vi "Extract IRF from PSED v2.vi"(6 "Termination Criteria":T1={"Max Iterations"=0, "Max Function Calls"=0, "Max Time"=1000.0, "Function Tolerance"=1e-06, "Parameter Tolerance"=1e-06, "Gradient Tolerance"=0.0, "Min Lambda"=1e-06, "Max Lambda"=1e-06, "Initial Tick Count"=0}, 8 "Error In":errorcluster, 9 "IRF*PSED Fixed Parameters":T7={"order"=0, "T"=0.0, "Time Constant Array"=[], "{S_k, C_k, phi_k, e_k} arrays"={"S_k Array"=[], "C_k Array"=[], "phi_k Array"=[], "e_k Array"=[]}, "IRF Extraction Options"={"Time Constant for IRF Extraction"=1e-18, "IRF Order"=0, "Fourier Series Smoothing"=enum."None", "Noise Threshold"=0.0, "Smoothing Width"=0.0, "Fourier Series Truncation"=enum."Automatic", "Truncation Order"=0, "Save Power Spectrum"=FALSE, "Smoothing"=FALSE, "Smoothing Parameter"=0.0, "Smoothing Order"=1, "Method"=enum."Direct"}} {"IRF Extraction Options"."Smoothing Order" min=1 max=10; "IRF Extraction Options"."Time Constant for IRF Extraction" format="%#_5g"}, 10 "Fit Settings":T2={"Use Original Plot # Points"=TRUE, "# Fit Plot Points"=0, "Fitting Method"=enum."Least Square", "Weighted Fit"=TRUE, "Show All Fit Components"=FALSE, "Axis Type"=0, "Show Fit Residuals"=TRUE, "Residual Type"=enum."Standard", "Fitting Algorithm"=enum."Levenberg-Marquardt"} {"Axis Type" items=["Linear", "Logarithmic"]}, 11 "Selected Plot Info":T12={"Multiplot XY Graph"=refnum, "Mouse Coordinates"={"Horizontal"=0, "Vertical"=0}, "Plot Index"=-1}) -> (0 "Error Out":errorcluster, 1 "Fit Result String":string, 2 "Power Spectrum":dbl[](array[numeric]), 3 "IRF Plot":cluster{"X Array":dbl[], "Y Array":dbl[]}, 5 "Smoothed Power Spectrum":dbl[](array[numeric]))   [LabVIEW 2021, in "Fits.lvlib"]
doc: "Extract IRF from provided decay and time constant"
uses:
  Fits.lvlib
  Graphs/XY Graph/XY Graph Selected Plot Info.ctl
  Graphs/XY Graph/XY Graph Refnum.ctl
  <vilib>/Utility/miscctls.llb/LVPoint32TypeDef.ctl
  IRF(X)PSED Fixed Parameters v3.ctl
  IRF(X)PSED Extraction Options.ctl
  Fourier Series Smoothing Option.ctl
  Fourier Series Truncation.ctl
  IRF Extraction Method.ctl
  Fit Settings.ctl
  Nonlinear Fit Method.ctl
  Ramp Type.ctl
  Residual Type.ctl
  Non-linear Fitting Algorithm.ctl
  My Fit Stopping Criteria.ctl
  Fit Plot Request Information.ctl
  <vilib>/Utility/miscctls.llb/LVPointDoubleTypeDef.ctl
  Fit Models.ctl
  D-Only Fixed Parameters.ctl
  Error/Error.lvlib
  Graphs/XY Graph/XY Graph Add-Ons.lvlib
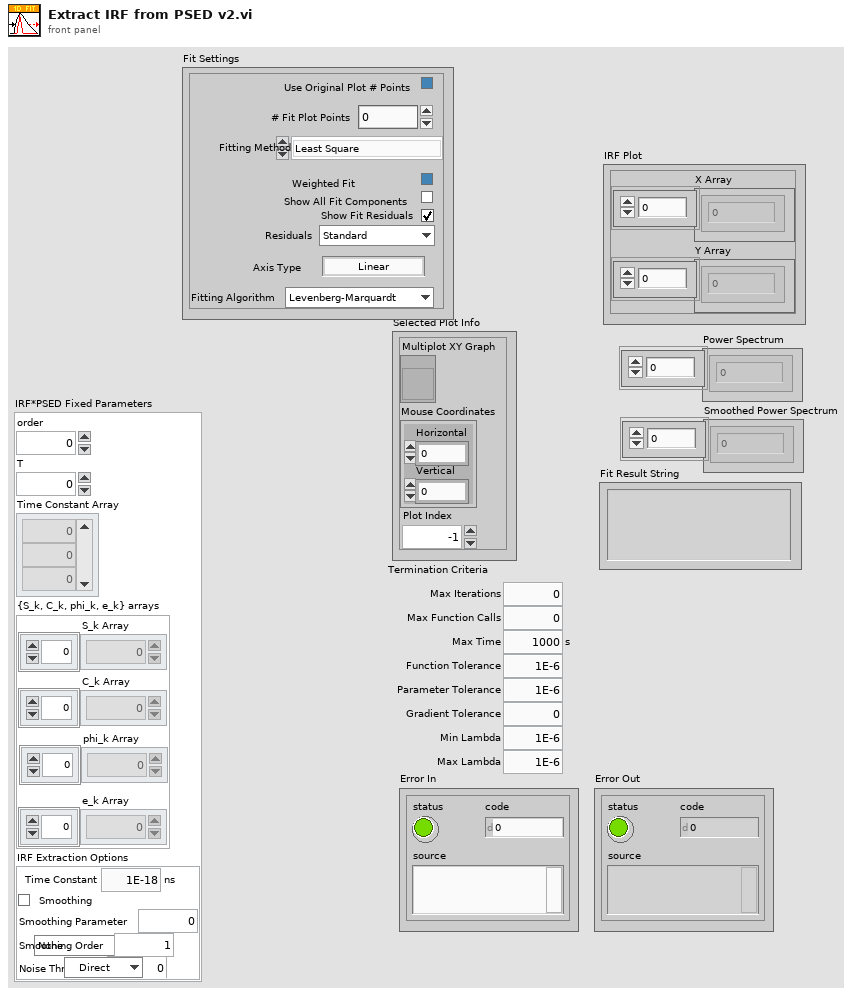
[diagram p1: front panel]
types:
  T1 = typedef "Fits.lvlib/My Fit Stopping Criteria.ctl" = cluster{"Max Iterations":i32, "Max Function Calls":i32, "Max Time":dbl[unit], "Function Tolerance":dbl, "Parameter Tolerance":dbl, "Gradient Tolerance":dbl, "Min Lambda":dbl, "Max Lambda":dbl, "Initial Tick Count":u32}
  T2 = typedef "Fits.lvlib/Fit Settings.ctl" = cluster{"Use Original Plot # Points":bool, "# Fit Plot Points":u32, "Fitting Method":T3, "Weighted Fit":bool, "Show All Fit Components":bool, "Axis Type":T4, "Show Fit Residuals":bool, "Residual Type":T5, "Fitting Algorithm":T6}
  T3 = typedef "Fits.lvlib/Nonlinear Fit Method.ctl" = enum16{"Least Square", "Least Absolute Residual", "Bisquare", "MLE"}
  T4 = typedef "Fits.lvlib/Ramp Type.ctl" = u16
  T5 = typedef "Fits.lvlib/Residual Type.ctl" = enum16{"Standard", "Normalized", "Reduced"}
  T6 = typedef "Fits.lvlib/Non-linear Fitting Algorithm.ctl" = enum16{"Levenberg-Marquardt", "Trust-Region Dogleg"}
  T7 = typedef "Fits.lvlib/IRF(X)PSED Fixed Parameters v3.ctl" = cluster{"order":i32, "T":dbl, "Time Constant Array":dbl[], "{S_k, C_k, phi_k, e_k} arrays":cluster{"S_k Array":dbl[], "C_k Array":dbl[], "phi_k Array":dbl[], "e_k Array":dbl[]}, "IRF Extraction Options":T8}
  T8 = typedef "Fits.lvlib/IRF(X)PSED Extraction Options.ctl" = cluster{"Time Constant for IRF Extraction":dbl[unit], "IRF Order":i32, "Fourier Series Smoothing":T9, "Noise Threshold":dbl, "Smoothing Width":dbl, "Fourier Series Truncation":T10, "Truncation Order":i32, "Save Power Spectrum":bool, "Smoothing":bool, "Smoothing Parameter":dbl, "Smoothing Order":u32, "Method":T11}
  T9 = typedef "Fits.lvlib/Fourier Series Smoothing Option.ctl" = enum16{"None", "Lanczos Factors", "Fejer Summation"}
  T10 = typedef "Fits.lvlib/Fourier Series Truncation.ctl" = enum16{"Automatic", "Fixed"}
  T11 = typedef "Fits.lvlib/IRF Extraction Method.ctl" = enum16{"Direct", "Topless", "Toeplitz"}
  T12 = typedef "XY Graph Add-Ons.lvlib/XY Graph Selected Plot Info.ctl" = cluster{"Multiplot XY Graph":T13, "Mouse Coordinates":T14, "Plot Index":i32}
  T13 = typedef "XY Graph Add-Ons.lvlib/XY Graph Refnum.ctl" = refnum<vi>
  T14 = typedef "LVPoint32TypeDef.ctl" = cluster{"Horizontal":i32, "Vertical":i32}
  T15 = typedef "Fits.lvlib/D-Only Fixed Parameters.ctl" = cluster{"Fix D-only Peak Location":bool, "Peak Location":dbl, "Fix D-only Peak FWHM":bool, "Peak FWHM":dbl}
  T16 = typedef "Fits.lvlib/Fit Plot Request Information.ctl" = cluster{"XY Graph Ref":refnum<vi>, "Mouse Coordinates":T17, "Fit Model":T18, "Plot Index":i32}
  T17 = typedef "LVPointDoubleTypeDef.ctl" = cluster{"X":dbl, "Y":dbl}
  T18 = typedef "Fits.lvlib/Fit Models.ctl" = enum16{"Select a Fit Model...", "           Single Peak", "Gaussian", "Asymmetric Gaussian", "Lorentzian", "Asymmetric Lorentzian", "Gaussian/Lorentzian", "Lorentzian/Gaussian", "           Double Peak", "Two Gaussians", "Two Asymmetric Gaussians", "Two H-Connected Gaussians", "Two T-Connected Gaussians", "Two H-Connected Asymmetric Gaussians", "Two T-Connected Asymmetric Gaussians", "           Triple Peak", "Three Gaussians", "Three Asymmetric Gaussians", "              Decays", "1-Exponential", "IRF*PSED", "2-Exponentials", "               ACF", "2D Gaussian ACF", "2D Gaussian + Blinking ACF", "2D Gaussian + Flow ACF", "3D Gaussian ACF", "3D Gaussian + Blinking ACF", "             Multiplot", "2D Gaussian ACF & 2D Gaussian + Flow ACF"}
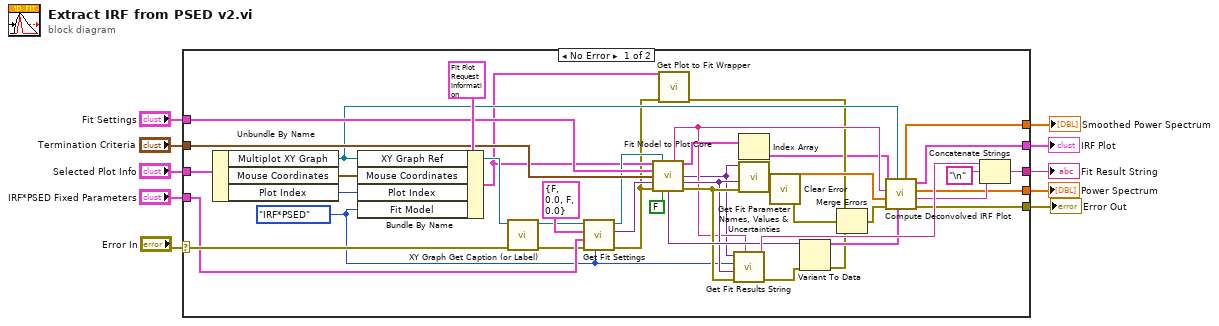
[diagram p0: block diagram]
diagram:
  n1 = case shown="No Error" "Error In" {
    selector: "Error In" -> [w51 w52]
    tunnel: [w46 w52] -> w10
    tunnel: "Selected Plot Info" -> [w17 _]
    tunnel: "IRF*PSED Fixed Parameters" -> [w38 _]
    tunnel: "Fit Settings" -> [w43 _]
    tunnel: [w42 _] -> w5
    tunnel: [w45 _] -> w4
    tunnel: "Termination Criteria" -> [w39 _]
    tunnel: [w35 _] -> w2
    tunnel: [w34 _] -> w1
    frame No Error {
      w23 = Fit_Models."IRF*PSED" ("Fit Model")
      n2 = Unbundle By Name(w17) -> ("Multiplot XY Graph"=w18:T13, "Mouse Coordinates"=w49:T14, "Plot Index"=w19:i32)
      n3 = Bundle By Name(cluster=T16 {"XY Graph Ref"=refnum, "Mouse Coordinates"={"X"=0.0, "Y"=0.0}, "Fit Model"=enum."Select a Fit Model...", "Plot Index"=-1} ("Fit Plot Information"), "XY Graph Ref"=w18, "Mouse Coordinates"=w49, "Plot Index"=w19, "Fit Model"=w23) -> (w16:T16)
      n4 = call "XY Graph Get Caption (or Label).vi"("error in (no error)"=w51, "XYGraph in"=w18) -> ("error out"=w31:errorcluster, "XYGraph out"=w30:T13)  [unwired: 7 in, 1 out]
      n5 = call "Get Fit Settings.vi"("Fit Model"=w23, "Error In"=w31, "Additional Parameters"=w38, "Fixed Parameters"=T15 {"Fix D-only Peak Location"=FALSE, "Peak Location"=0.0, "Fix D-only Peak FWHM"=FALSE, "Peak FWHM"=0.0}, "XY Graph Ref"=w30) -> ("Error Out"=w15:errorcluster, "Additional Fit Settings"=w28:variant, "LM Function & Gradient"=w26:refnum<vi>)  [unwired: 4 in]
      n6 = call "Fit Model to Plot Core.vi"("Fit Plot Information"=w16, "LM Function & Gradient"=w26, "Fit Settings"=w43, "Termination Criteria"=w39, "Additional Data (in)"=w28, "error in (no error)"=w15, "Send Graph to Notebook?"=FALSE ("Send Graph to Notebook? (F)")) -> ("Plot Name"=w22:string, "Array of Plots (Fit, Components, Residuals)"=w24:cluster{"X Array":dbl[], "Y Array":dbl[]}[], "Fit Parameters Cluster"=w21:variant, "Fit Parameters Uncertainties Cluster"=w25:variant, "Additional Data (out)"=w37:variant, "error out"=w29:errorcluster)  [unwired: 1 in, 2 out]
      n7 = call "Get Plot to Fit Wrapper.vi"("error in (no error)"=w15, "Fit Plot Information"=w16) -> ("error out"=w14:errorcluster)  [unwired: 4 in, 5 out]
      n8 = call "Get Fit Results String.vi"("Plot Name"=w22, "error in (no error)"=w29, "Fit Parameters Uncertainties Cluster"=w25, "Fit Model"=w23, "Fit Parameters Cluster"=w21) -> ("error out"=w20:errorcluster, "Fit Results String"=w47:string)  [unwired: 5 in]
      n9 = Index Array(array=w24) -> (element=w13:cluster{"X Array":dbl[], "Y Array":dbl[]})  [unwired: 1 in]
      n10 = call "Get Fit Parameter Names, Values & Uncertainties.vi"("error in (no error)"=w29, "Fit Parameter Uncertainties"=w25, "Fit Parameters"=w21) -> ("Error Out"=w27:errorcluster, "Fit Parameter Values"=w44:dbl[])  [unwired: 5 in, 2 out]
      n11 = call "Clear Error.vi"("Error In"=w27) -> ("no Error Out"=w11:errorcluster)  [unwired: 8 in]
      n12 = Variant To Data(error in=w20, Variant=w37) -> (data=w36:T7, error out=w33:errorcluster)  [unwired: 1 in]
      n13 = Merge Errors(w14, w11, w33) -> (w12:errorcluster)
      n14 = call "Compute Deconvolved IRF Plot.vi"("IRF*PSED fixed Parameters"=w36, "XYGraph in"=w18, "error in (no error)"=w12, "Fit Parameter Values"=w44, "Plot Name"=w22, "Fitted Decay"=w13) -> ("error out"=w46:errorcluster, "Amplitude String"=w41:string, "Power Spectrum"=w35:dbl[], "IRF Plot"=w45:cluster{"X Array":dbl[], "Y Array":dbl[]}, "Smoothed Power Spectrum"=w34:dbl[])  [unwired: 1 in]
      n15 = Concatenate Strings(w47, "\n" ("string"), w41) -> (w42:string)
    }
    frame Error {
    }
  }
  "Error Out" <- w10
  "Fit Result String" <- w5
  "IRF Plot" <- w4
  "Power Spectrum" <- w2
  "Smoothed Power Spectrum" <- w1
